vi "_RT Read XML Lens.vi"(4 "error in":errorcluster, 7 "XML String":string) -> (0 "error out":errorcluster, 1 "Lens":T1[](array[typedef]) {"Value" format="%#.6g"}, 3 "Remaining String":string)   [LabVIEW 2015]
uses:
  Type/_XML Lens.ctl
  Type/_XML Type.ctl
  Server/_Server Global.vi
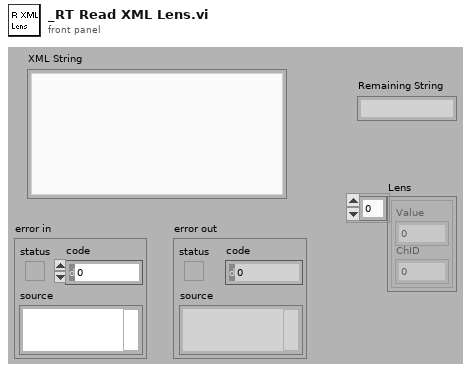
[diagram p1: front panel]
types:
  T1 = typedef "_XML Lens.ctl" = cluster{"Value":dbl, "ChID":u8}
  T2 = typedef "_XML Type.ctl" = enum16{"Configuration", "ConTable", "Method", "Experiment", "Mass Range", "Table", "LensTable", "ParamTable", "TuneParam", "MetParam", "MassRange", "LCMethod", "LCMethodFile", "RackType", "Vial", "PlatePos", "InjVol"}
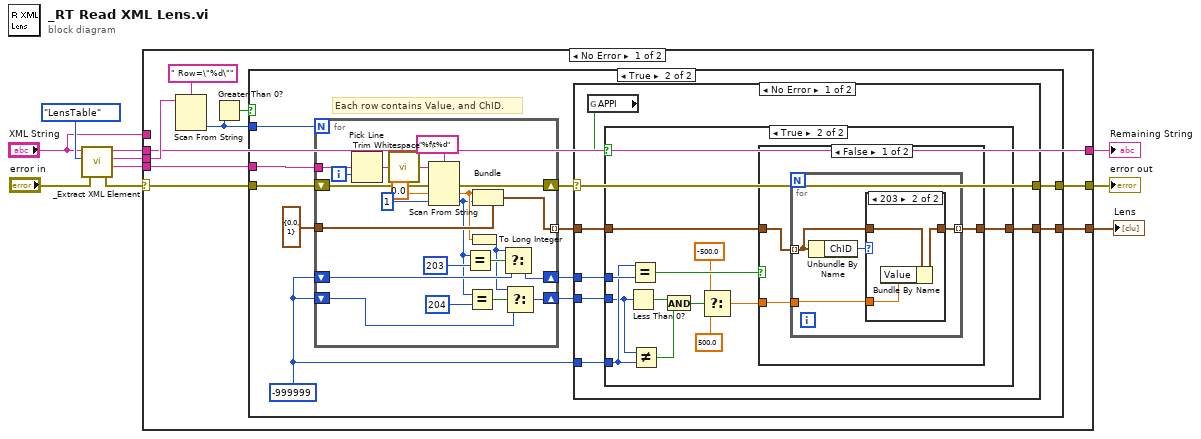
[diagram p0: block diagram]
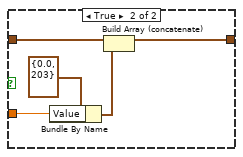
[diagram p5: hidden frame]
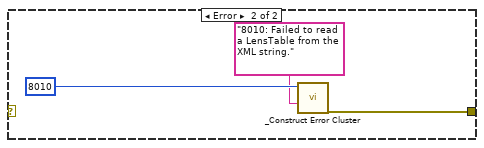
[diagram p6: hidden frame]
diagram:
  n1 = call "_Extract XML Element.vi"("error in"="error in", "XML Type"=_XML_Type."LensTable", "XML String"="XML String") -> ("error out"=w7:errorcluster, "Element"=w6:string, "Attributes"=w5:string, "Remaining String"=w4:string)  [unwired: 1 out]
  n2 = case shown="No Error" w7 {
    selector: w7 -> [w12 w93]
    tunnel: [w16 w93] -> w10
    tunnel: w6 -> [w17 _]
    tunnel: w5 -> [w18 _]
    tunnel: w4 -> [w15 _]
    tunnel: "XML String" -> [_ w92]
    tunnel: [w15 w92] -> w2
    tunnel: [w11 _] -> w1
    frame No Error {
      n3 = Scan From String(format string=" Row=\"%d\"", input string=w18) -> (output 1=w13:i32)  [unwired: 2 in, 4 out]
      n4 = Greater Than 0?(x=w13) -> (x > 0?=w14:bool)
      n5 = case shown="True" w14 {
        tunnel: w13 -> [_ w30]
        tunnel: w17 -> [_ w29]
        tunnel: [_ w25] -> w16
        tunnel: w12 -> [_ w27]
        tunnel: [_ w23] -> w11
        frame False {
        }
        frame True {
          w20 = -999999 ("Value")
          # "Each row contains Value, and ChID."
          n6 = for {
            N: w30 -> [_]
            tunnel: w29 -> [w89]
            shift-right: [w86] -> w26
            shift-left: w27 -> [w85]
            tunnel: [w84] -> w24 mode=indexing
            tunnel: T1 {"Value"=0.0, "ChID"=1} ("Lens") -> [w82]
            shift-right: [w77] -> w22
            shift-left: w20 -> [w78]
            shift-right: [w74] -> w21
            shift-left: w20 -> [w72]
            i -> [w88]
            n7 = Pick Line(multi-line string=w89, line index=w88) -> (output string=w90:string)  [unwired: 1 out]
            n8 = call <vilib>:"Trim Whitespace.vi"("string"=w90) -> ("trimmed string"=w87:string)  [unwired: 1 in]
            n9 = Scan From String(format string="%f\t%d", input string=w87, error in=w85, default 1=0.0 ("Ch#"), default 2=u8 1 ("Ch#")) -> (error out=w86:errorcluster, output 1=w73:dbl, output 2=w71:u8)  [unwired: 1 in, 2 out]
            n10 = Equal?(x=w71, y=u8 203) -> (x = y?=w79:bool)
            n11 = Equal?(x=w71, y=u8 204) -> (x = y?=w76:bool)
            n12 = To Long Integer(number=w73) -> (32bit integer=w70:i32)
            n13 = Bundle(cluster=w82, "Value"=w73, "ChID"=w71) -> (w84:T1)
            n14 = Select(t=w70, s=w79, f=w78) -> (s? t:f=w77:i32)
            n15 = Select(t=w70, s=w76, f=w72) -> (s? t:f=w74:i32)
          }
          n16 = case shown="No Error" w26 {
            selector: w26 -> [w37 _]
            tunnel: [w37 w68] -> w25
            tunnel: w24 -> [w35 _]
            tunnel: [w34 _] -> w23
            tunnel: w22 -> [w33 _]
            tunnel: w21 -> [w32 _]
            tunnel: w20 -> [w31 _]
            frame No Error {
              n17 = global read "_Server Global.vi" "APPI"() -> (w36:bool)
              n18 = case shown="True" w36 {
                tunnel: w35 -> [w38 w49]
                tunnel: [w38 w39] -> w34
                tunnel: w33 -> [_ w48]
                tunnel: w32 -> [_ w46]
                tunnel: w31 -> [_ w47]
                frame False {
                }
                frame True {
                  n19 = Less Than 0?(x=w46) -> (x < 0?=w45:bool)
                  n20 = Equal?(x=w47, y=w48) -> (x = y?=w50:bool)
                  n21 = Not Equal?(x=w46, y=w47) -> (x != y?=w44:bool)
                  n22 = And(x=w45, y=w44) -> (x .and. y?=w43:bool)
                  n23 = Select(t=-500.0, s=w43, f=500.0 ("t")) -> (s? t:f=w40:dbl)
                  n24 = case shown="False" w50 {
                    tunnel: w49 -> [w53 w66]
                    tunnel: [w52 w65] -> w39
                    tunnel: w40 -> [w51 w63]
                    frame False {
                      n25 = for {
                        tunnel: w53 -> [w56] mode=indexing
                        tunnel: w51 -> [w54]
                        tunnel: [w55] -> w52 mode=indexing
                        n26 = Unbundle By Name(w56) -> ("ChID"=w57:u8)
                        n27 = case shown="203" w57 {
                          tunnel: w56 -> [w58 w61]
                          tunnel: [w58 w60] -> w55
                          tunnel: w54 -> [_ w59]
                          frame 0, Default {
                          }
                          frame 203 {
                            n28 = Bundle By Name(cluster=w61, "Value"=w59) -> (w60:T1)
                          }
                        }
                      }
                    }
                    frame True {
                      n29 = Bundle By Name(cluster=T1 {"Value"=0.0, "ChID"=203} ("Lens"), "Value"=w63) -> (w62:T1)
                      n30 = Build Array (concatenate)(w66, w62) -> (w65:T1[])
                    }
                  }
                }
              }
            }
            frame Error {
              n31 = call "_Construct Error Cluster.vi"("reason"="8010: Failed to read a LensTable from the XML string.", "errorCode"=8010) -> ("error out"=w68:errorcluster)  [unwired: 2 in, 3 out]
            }
          }
        }
      }
    }
    frame Error {
    }
  }
  "error out" <- w10
  "Remaining String" <- w2
  "Lens" <- w1
